vi "_FPGA_SelfInitStrobe.vi"(3 "Stop_strobe_in":bool) -> (0 "Init_strobe_out":bool, 1 "State_out":bool)   [LabVIEW 2018]
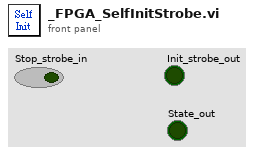
[diagram p1: front panel]
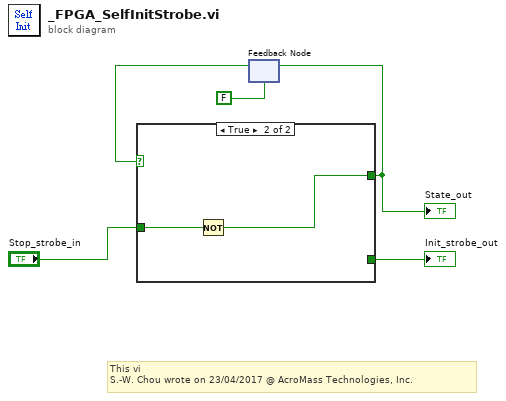
[diagram p0: block diagram]
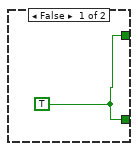
[diagram p2: hidden frame]
diagram:
  # "This vi  \nS.-W. Chou wrote on 23/04/2017 @ AcroMass Technologies, Inc."
  n1 = feedback #1(FALSE) -> (w5:bool)
  n2 = case shown="True" w5 {
    tunnel: "Stop_strobe_in" -> [_ w8]
    tunnel: [w6 _] -> w2
    tunnel: [w6 w7] -> w1
    frame False {
      w6 = TRUE
    }
    frame True {
      n3 = Not(x=w8) -> (.not. x?=w7:bool)
    }
  }
  "Init_strobe_out" <- w2
  "State_out" <- w1
  n4 = feedback-in #1(w1) -> ()
